vi "read connection message.vi"(8 "error in":errorcluster, 11 "data":variant) -> (0 "error out":errorcluster, 3 "conn":refnum<class "connection maintainer.lvclass">)   [LabVIEW 2015, in "connection maintainer.lvclass"]
uses:
  connection maintainer.lvclass
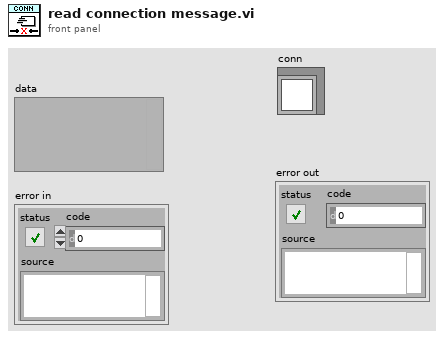
[diagram p1: front panel]
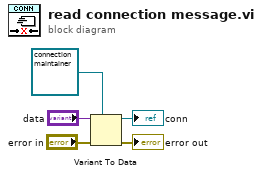
[diagram p0: block diagram]
diagram:
  n1 = Variant To Data(error in="error in", type=refnum<class "connection maintainer.lvclass"> refnum ("new connection"), Variant="data") -> (data=→"conn":refnum<class "connection maintainer.lvclass">, error out=→"error out":errorcluster)
